vi "-8770 Source empty--error.vi"(8 "error in":errorcluster) -> (0 "error out":errorcluster)   [LabVIEW 2025, in "Config from EXCEL.lvclass"]
uses:
  Config from EXCEL.lvclass
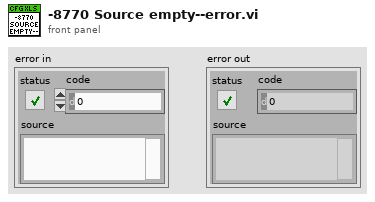
[diagram p1: front panel]
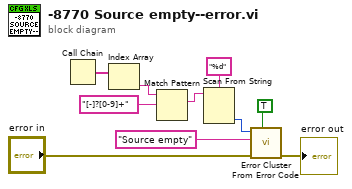
[diagram p0: block diagram]
diagram:
  n1 = Call Chain() -> (call chain=w6:string[])
  n2 = Index Array(array=w6) -> (element=w4:string)  [unwired: 1 in]
  n3 = Match Pattern(string=w4, regular expression="[-]?[0-9]+") -> (match substring=w3:string)  [unwired: 1 in, 3 out]
  n4 = Scan From String(format string="%d", input string=w3) -> (output 1=w1:i32)  [unwired: 3 in, 3 out]
  n5 = call <vilib>:"Error Cluster From Error Code.vi"("show call chain? (False)"=TRUE, "error in (no error)"="error in", "error message (\"\")"="Source empty" ("error message (\"\")"), "error code (0)"=w1) -> ("error out"=→"error out":errorcluster)  [unwired: 5 in]
